vi "Channel_Detect.vi"() -> ()   [LabVIEW 2024]
uses:
  <vilib>/DAQmx/create/channels.llb/DAQmx Create Channel (AO-Voltage-Basic).vi
panel:
  in  "Connect":bool
  out "error out":errorcluster
  in  "physical channels":tag
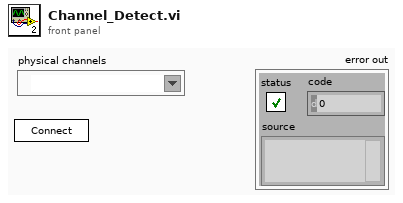
[diagram p1: front panel]
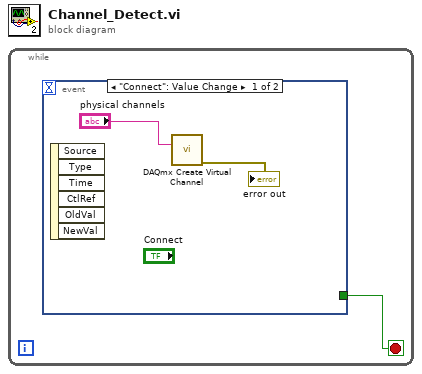
[diagram p0: block diagram]
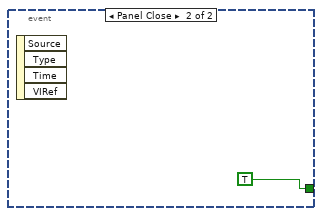
[diagram p2: hidden frame]
diagram:
  n1 = while {
    stop <- w1 stop-if-true
    n2 = event shown="[0] \"Connect\": Value Change" {
      selector: _ -> [_ _]
      dyn-events: _ -> [_ _]
      timeout: _ -> [_ _]
      tunnel: [_ TRUE] -> w1
      event "Connect": Value Change {
        n3 = event-data() -> ()  [unwired: 1 in, 6 out]
        n4 = call-poly <vilib>:"DAQmx Create Virtual Channel.vi"("physical channels"="physical channels") -> ("error out"=→"error out":errorcluster)  [unwired: 13 in, 1 out]
      }
      event Panel Close {
        n5 = event-data() -> ()  [unwired: 1 in, 4 out]
      }
    }
  }
